vi "Delay Basicdata inquiry.vi"(7 "Channel  (1: CH1)":u16(ring)=1 items=["CH1"=1, "CH2"=2, "CH3"=3, "CH4"=4], 8 "error in (no error)":errorcluster, 11 "VISA resource name":refnum<visa-resource-name>) -> (0 "error out":errorcluster, 1 "Start":dbl, 2 "Cycles":dbl, 3 "VISA resource name out":refnum<visa-resource-name>, 4 "End State":string, 6 "Groups":dbl)   [LabVIEW 2020, in "GPP.lvlib"]
uses:
  GPP.lvlib
  Function/VISA_COMMON.ctl
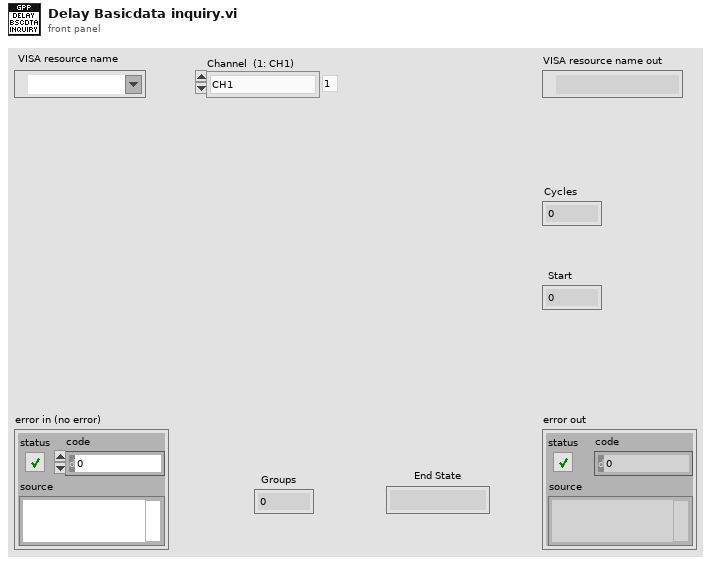
[diagram p1: front panel]
types:
  T1 = typedef "GPP.lvlib/VISA_COMMON.ctl" = enum16{"Initial", "Write CMD", "Read Result", "Read History", "Close"}
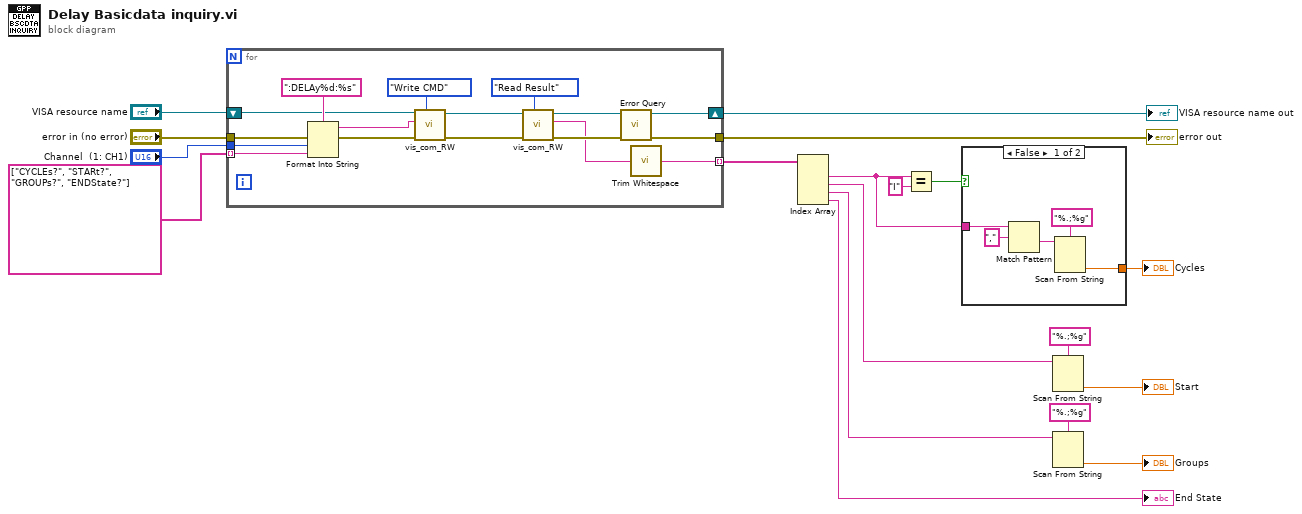
[diagram p0: block diagram]
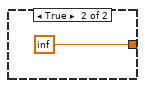
[diagram p2: hidden frame]
diagram:
  n1 = for {
    tunnel: "error in (no error)" -> [w29]
    tunnel: "Channel  (1: CH1)" -> [w27]
    tunnel: string[] ["CYCLEs?", "STARt?", "GROUPs?", "ENDState?"] -> [w24] mode=indexing
    tunnel: [w25] -> w5
    tunnel: [w21] -> w14 mode=indexing
    shift-right: [w19] -> w4
    shift-left: "VISA resource name" -> [w23]
    n2 = Format Into String(format string=":DELAy%d:%s", error in=w29, w27, w24) -> (resulting string=w22:string, error out=w28:errorcluster)  [unwired: 1 in]
    n3 = call "vis_com_RW.vi"("Funciton"=VISA_COMMON."Write CMD", "error in (no error)"=w28, "CMD String"=w22, "VISA resource in"=w23) -> ("error out"=w33:errorcluster, "VISA resource out"=w32:refnum<visa-resource-name>)  [unwired: 5 in, 1 out]
    n4 = call "vis_com_RW.vi"("Funciton"=VISA_COMMON."Read Result", "error in (no error)"=w33, "VISA resource in"=w32) -> ("error out"=w30:errorcluster, "Result"=w20:string, "VISA resource out"=w31:refnum<visa-resource-name>)  [unwired: 6 in]
    n5 = call "Error Query.vi"("error in (no error)"=w30, "VISA resource name"=w31) -> ("error out"=w25:errorcluster, "VISA resource name out"=w19:refnum<visa-resource-name>)  [unwired: 6 in, 2 out]
    n6 = call <vilib>:"Trim Whitespace.vi"("string"=w20) -> ("trimmed string"=w21:string)  [unwired: 1 in]
  }
  "error out" <- w5
  "VISA resource name out" <- w4
  n7 = Index Array(array=w14) -> (element #1=w1:string, element #2=w11:string, element #3=w10:string, element #4=→"End State":string)  [unwired: 4 in]
  n8 = Equal?(x=w1, y="I") -> (x = y?=w3:bool)
  n9 = case shown="False" w3 {
    tunnel: [w37 inf ("t")] -> w2
    tunnel: w1 -> [w36 _]
    frame False {
      n10 = Match Pattern(string=w36, regular expression=",") -> (after substring=w38:string)  [unwired: 1 in, 3 out]
      n11 = Scan From String(format string="%.;%g", input string=w38) -> (output 1=w37:dbl)  [unwired: 3 in, 3 out]
    }
    frame True {
    }
  }
  "Cycles" <- w2
  n12 = Scan From String(format string="%.;%g", input string=w11) -> (output 1=→"Start":dbl)  [unwired: 3 in, 3 out]
  n13 = Scan From String(format string="%.;%g", input string=w10) -> (output 1=→"Groups":dbl)  [unwired: 3 in, 3 out]
